vi "Specified environment does not exist--error.vi"() -> (0 "error out":errorcluster)   [LabVIEW 2025]
doc: "Indicates that the specified executable path does not point to an existing file. This error is raised before process execution to prevent attempting to start a non-existent program."
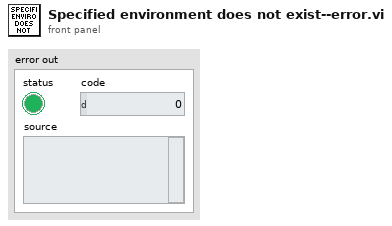
[diagram p1: front panel]
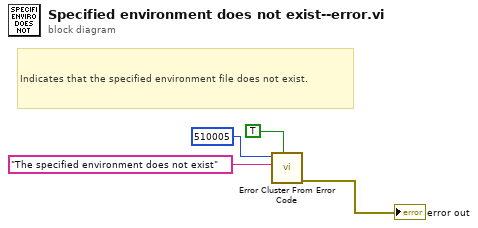
[diagram p0: block diagram]
diagram:
  # "Indicates that the specified environment file does not exist."
  n1 = call <vilib>:"Error Cluster From Error Code.vi"("show call chain? (False)"=TRUE, "error message (\"\")"="The specified environment does not exist" ("error message (\"\")"), "error code (0)"=510005) -> ("error out"=→"error out":errorcluster)  [unwired: 6 in]
